vi "TTA_Draw_Labelled_Rectangle.vi"(6 "color(black)":u32(colorbox), 7 "oval dimension":i16, 8 "error in":errorcluster, 9 "Dimensions":T1, 10 "Label":string, 11 "picture":picture) -> (0 "error out":errorcluster, 3 "2D Picture\nOut":picture)   [LabVIEW 2016]
uses:
  <vilib>/Analysis/baseanly.llb/Mean (DBL).vi
  <vilib>/Analysis/NI_AALBase.lvlib
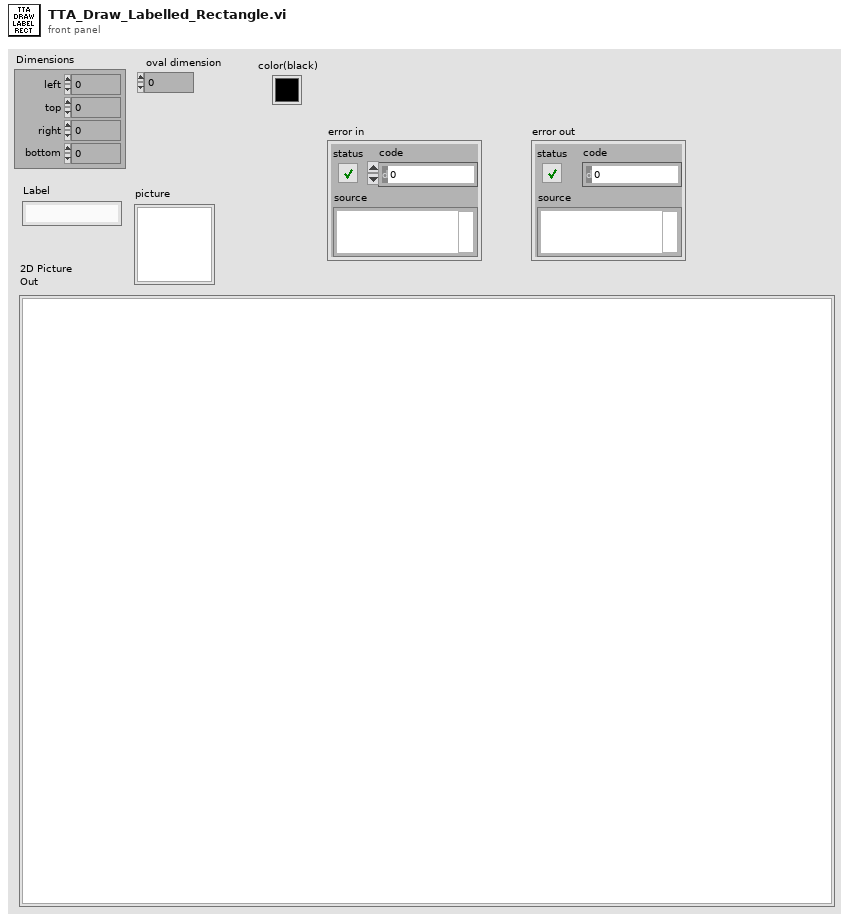
[diagram p1: front panel]
types:
  T1 = cluster{"left":i16, "top":i16, "right":i16, "bottom":i16}
  T2 = enum16{"User-specified Font", "Application Font", "System Font", "Dialog Font"}
  T3 = cluster{"Font Name:":string, "Size":i16, "Strikeout?":bool, "Italic?":bool, "Underline?":bool, "Outline?":bool, "Shadow?":bool, "Bold?":bool}
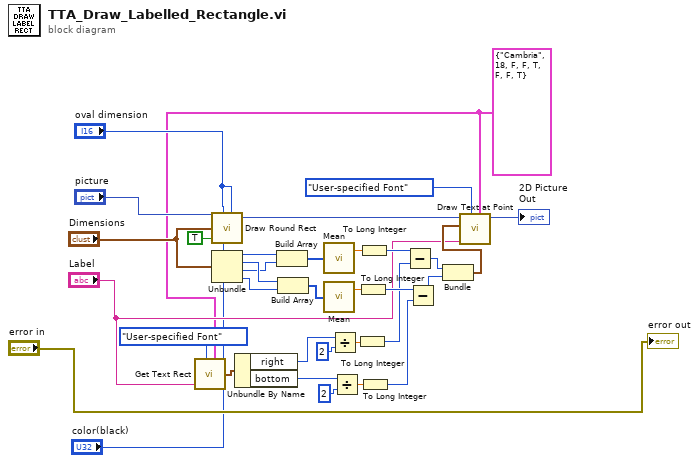
[diagram p0: block diagram]
diagram:
  w3 = T3 {"Font Name:"="Cambria", "Size"=18, "Strikeout?"=FALSE, "Italic?"=FALSE, "Underline?"=TRUE, "Outline?"=FALSE, "Shadow?"=FALSE, "Bold?"=TRUE} ("[user-specified font]")
  n1 = call <vilib>:"Get Text Rect.vi"("desired font(Application)"=T2."User-specified Font", "text"="Label", "[user-specified font]"=w3) -> ("rect"=w11:T1)  [unwired: 6 in]
  n2 = call <vilib>:"Draw Round Rect.vi"("picture"="picture", "oval width"="oval dimension", "rect"="Dimensions", "fill?(F)"=TRUE, "color(black)"="color(black)", "oval height"="oval dimension") -> ("new picture"=w30:picture)  [unwired: 3 in]
  n3 = Unbundle("Dimensions") -> ("left"=w18:i16, "top"=w20:i16, "right"=w19:i16, "bottom"=w21:i16)
  n4 = Unbundle By Name(w11) -> ("right"=w12:i16, "bottom"=w15:i16)
  n5 = Build Array(w18, w19) -> (w22:i16[])
  n6 = Build Array(w20, w21) -> (w23:i16[])
  n7 = call-poly <vilib>:"Mean.vi"("X"=w22) -> ("mean"=w24:dbl)  [unwired: 1 out]
  n8 = call-poly <vilib>:"Mean.vi"("X"=w23) -> ("mean"=w25:dbl)  [unwired: 1 out]
  n9 = Divide(x=w12, y=i16 2) -> (x/y=w16:dbl)
  n10 = Divide(x=w15, y=i16 2) -> (x/y=w17:dbl)
  n11 = To Long Integer(number=w16) -> (32bit integer=w27:i32)
  n12 = To Long Integer(number=w25) -> (32bit integer=w28:i32)
  n13 = To Long Integer(number=w24) -> (32bit integer=w26:i32)
  n14 = To Long Integer(number=w17) -> (32bit integer=w29:i32)
  n15 = Subtract(x=w26, y=w27) -> (x-y=w31:i32)
  n16 = Subtract(x=w28, y=w29) -> (x-y=w32:i32)
  n17 = Bundle(w31, w32) -> (w33:cluster{i32, i32})  [unwired: 1 in]
  n18 = call <vilib>:"Draw Text at Point.vi"("[user-specified font]"=w3, "desired font(Application)"=T2."User-specified Font", "text"="Label", "origin"=w33, "picture"=w30) -> ("new picture"=→"2D Picture\nOut":picture)  [unwired: 5 in, 1 out]
  "error out" <- "error in"
